vi "Sub01_CommandBuilder.vi"(8 "error in (no error)":errorcluster, 9 "CommandInfo":T1={"RedBall"={"Min"={"G"=0, "B"=0, "R"=160}, "Max"={"G"=160, "B"=160, "R"=255}}, "YellowBall"={"Min"={"G"=140, "B"=0, "R"=140}, "Max"={"G"=255, "B"=175, "R"=255}}, "WhiteBall"={"Min"={"G"=100, "B"=100, "R"=100}, "Max"={"G"=255, "B"=255, "R"=255}}, "BallDiameter"=11, "BackGround"={"Min"={"G"=91, "B"=202, "R"=39}, "Max"={"G"=116, "B"=255, "R"=62}}, "Border"={"Min"={"G"=0, "B"=121, "R"=0}, "Max"={"G"=42, "B"=126, "R"=14}}}, 10 "filenames":string[](array[string]), 11 "path in":path) -> (0 "error out":errorcluster, 3 "String":string)   [LabVIEW 2019]
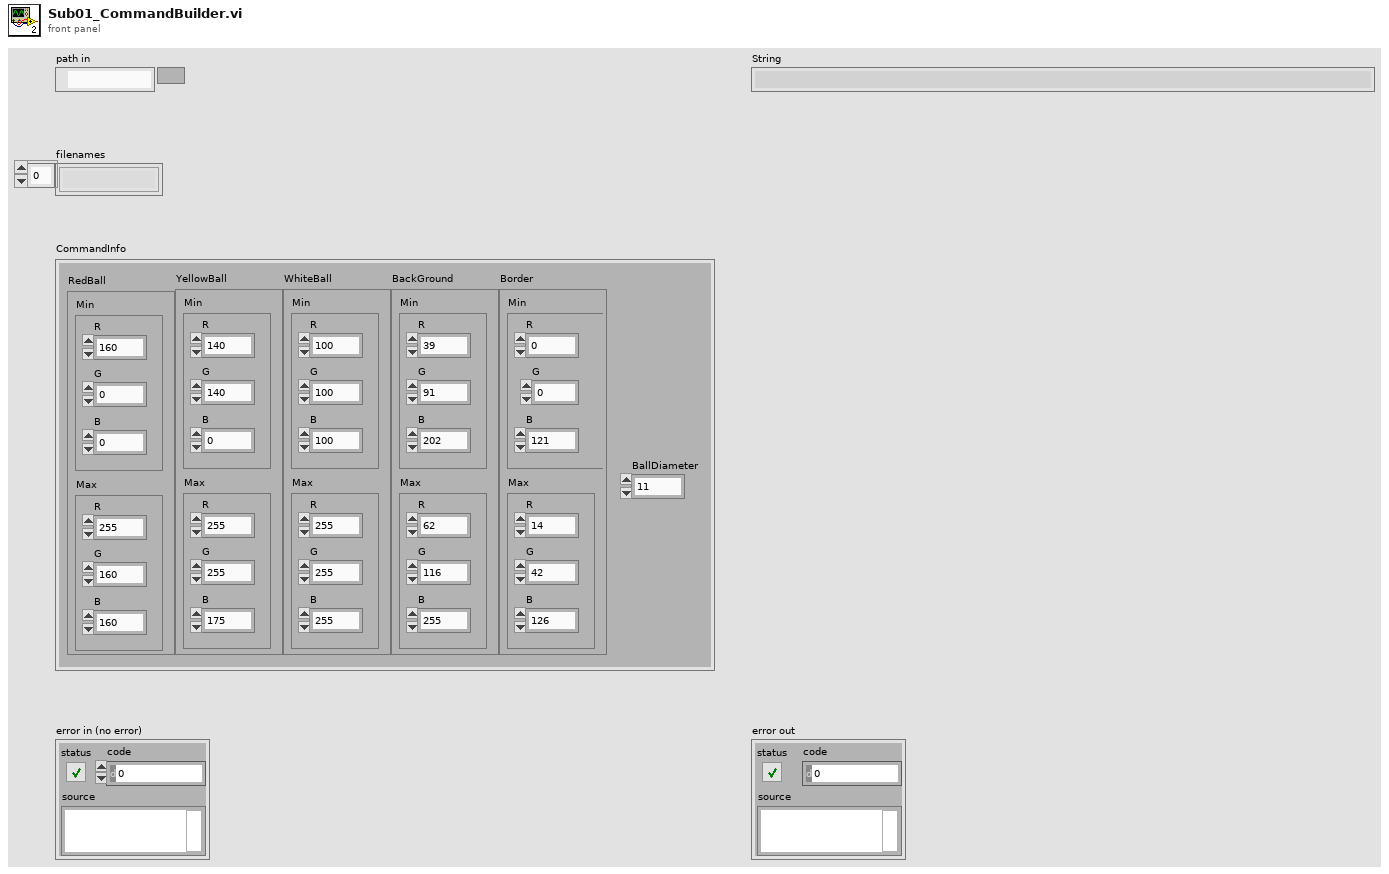
[diagram p1: front panel]
types:
  T1 = cluster{"RedBall":cluster{"Min":cluster{"G":u32, "B":u32, "R":u32}, "Max":cluster{"G":u32, "B":u32, "R":u32}}, "YellowBall":cluster{"Min":cluster{"G":u32, "B":u32, "R":u32}, "Max":cluster{"G":u32, "B":u32, "R":u32}}, "WhiteBall":cluster{"Min":cluster{"G":u32, "B":u32, "R":u32}, "Max":cluster{"G":u32, "B":u32, "R":u32}}, "BallDiameter":u32, "BackGround":cluster{"Min":cluster{"G":u32, "B":u32, "R":u32}, "Max":cluster{"G":u32, "B":u32, "R":u32}}, "Border":cluster{"Min":cluster{"G":u32, "B":u32, "R":u32}, "Max":cluster{"G":u32, "B":u32, "R":u32}}}
  T2 = typedef "imagedata.ctl" = cluster{"image type":i32, "image depth":i32, "image":u8[], "mask":u8[], "colors":u32[], "Rectangle":cluster{"left":i16, "top":i16, "right":i16, "bottom":i16}}
  T3 = cluster{"Min":cluster{"G":u32, "B":u32, "R":u32}, "Max":cluster{"G":u32, "B":u32, "R":u32}}
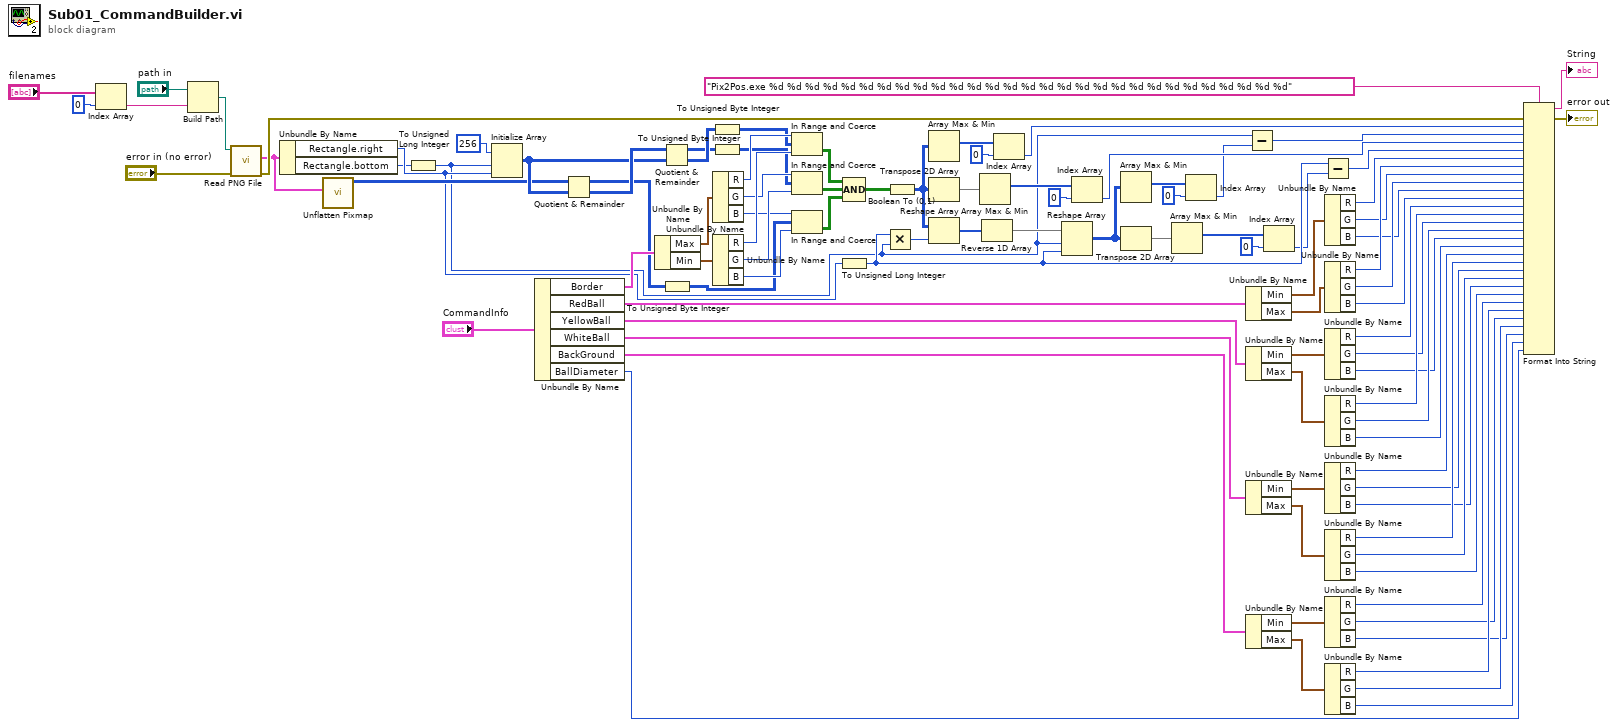
[diagram p0: block diagram]
diagram:
  n1 = Index Array(array="filenames", index=0) -> (element=w32:string)
  n2 = Build Path(base path="path in", name or relative path=w32) -> (appended path=w93:path)
  n3 = call <vilib>:"Read PNG File.vi"("error in (no error)"="error in (no error)", "path to PNG file"=w93) -> ("error out"=w94:errorcluster, "image data"=w30:T2)  [unwired: 7 in, 1 out]
  n4 = Unbundle By Name(w30) -> ("Rectangle.right"=w18:i16, "Rectangle.bottom"=w17:i16)
  n5 = call <vilib>:"Unflatten Pixmap.vi"("image data"=w30) -> ("24-bit pixmap"=w31:u32[][])  [unwired: 4 in, 6 out]
  n6 = To Unsigned Long Integer(number=w17) -> (unsigned 32bit integer=w7:u32)
  n7 = Initialize Array(u32 256 ("element"), w7, w18) -> (w37:u32[][])
  n8 = Unbundle By Name("CommandInfo") -> ("Border"=w50:T3, "RedBall"=w88:T3, "YellowBall"=w81:T3, "WhiteBall"=w80:T3, "BackGround"=w71:T3, "BallDiameter"=w49:u32)
  n9 = Quotient & Remainder(x=w31, y=w37) -> (x-y*floor(x/y)=w44:u32[][], floor(x/y)=w47:u32[][])
  n10 = Unbundle By Name(w50) -> ("Max"=w52:cluster{"G":u32, "B":u32, "R":u32}, "Min"=w51:cluster{"G":u32, "B":u32, "R":u32})
  n11 = Quotient & Remainder(x=w47, y=w37) -> (x-y*floor(x/y)=w45:u32[][], floor(x/y)=w46:u32[][])
  n12 = To Unsigned Byte Integer(number=w44) -> (unsigned 8bit integer=w36:u8[][])
  n13 = To Unsigned Byte Integer(number=w46) -> (unsigned 8bit integer=w34:u8[][])
  n14 = To Unsigned Byte Integer(number=w45) -> (unsigned 8bit integer=w35:u8[][])
  n15 = Unbundle By Name(w52) -> ("R"=w43:u32, "G"=w41:u32, "B"=w39:u32)
  n16 = Unbundle By Name(w51) -> ("R"=w42:u32, "G"=w40:u32, "B"=w38:u32)
  n17 = In Range and Coerce(upper limit=w43, x=w34, lower limit=w42) -> (In Range?=w29:bool[][])  [unwired: 1 out]
  n18 = In Range and Coerce(upper limit=w41, x=w35, lower limit=w40) -> (In Range?=w28:bool[][])  [unwired: 1 out]
  n19 = In Range and Coerce(upper limit=w39, x=w36, lower limit=w38) -> (In Range?=w27:bool[][])  [unwired: 1 out]
  n20 = To Unsigned Long Integer(number=w18) -> (unsigned 32bit integer=w8:u32)
  n21 = Compound Arithmetic op=AND(w29, w28, w27) -> (w26:bool[][])
  n22 = Multiply(x=w8, y=w7) -> (x*y=w25:u32)
  n23 = Boolean To (0,1)(Boolean=w26) -> (0, 1=w20:i16[][])
  n24 = Array Max & Min(array=w20) -> (max index (indices)=w12:i32[])  [unwired: 3 out]
  n25 = Transpose 2D Array(2D array=w20) -> (transposed array=w23:i16[][])
  n26 = Reshape Array(w20, w25) -> (w21:i16[])
  n27 = Array Max & Min(array=w23) -> (max index (indices)=w11:i32[])  [unwired: 3 out]
  n28 = Reverse 1D Array(array=w21) -> (reversed array=w24:i16[])
  n29 = Index Array(array=w12, index=0) -> (element=w6:i32)
  n30 = Reshape Array(w24, w7, w8) -> (w19:i16[][])
  n31 = Index Array(array=w11, index=0) -> (element=w5:i32)
  n32 = Array Max & Min(array=w19) -> (max index (indices)=w9:i32[])  [unwired: 3 out]
  n33 = Transpose 2D Array(2D array=w19) -> (transposed array=w22:i16[][])
  n34 = Array Max & Min(array=w22) -> (max index (indices)=w10:i32[])  [unwired: 3 out]
  n35 = Index Array(array=w9, index=0) -> (element=w4:i32)
  n36 = Unbundle By Name(w88) -> ("Min"=w87:cluster{"G":u32, "B":u32, "R":u32}, "Max"=w86:cluster{"G":u32, "B":u32, "R":u32})
  n37 = Unbundle By Name(w81) -> ("Min"=w85:cluster{"G":u32, "B":u32, "R":u32}, "Max"=w84:cluster{"G":u32, "B":u32, "R":u32})
  n38 = Unbundle By Name(w80) -> ("Min"=w83:cluster{"G":u32, "B":u32, "R":u32}, "Max"=w82:cluster{"G":u32, "B":u32, "R":u32})
  n39 = Unbundle By Name(w71) -> ("Min"=w73:cluster{"G":u32, "B":u32, "R":u32}, "Max"=w72:cluster{"G":u32, "B":u32, "R":u32})
  n40 = Subtract(x=w7, y=w4) -> (x-y=w3:u32)
  n41 = Index Array(array=w10, index=0) -> (element=w2:i32)
  n42 = Subtract(x=w8, y=w2) -> (x-y=w1:u32)
  n43 = Unbundle By Name(w87) -> ("R"=w79:u32, "G"=w77:u32, "B"=w75:u32)
  n44 = Unbundle By Name(w86) -> ("R"=w78:u32, "G"=w76:u32, "B"=w74:u32)
  n45 = Unbundle By Name(w85) -> ("R"=w70:u32, "G"=w68:u32, "B"=w66:u32)
  n46 = Unbundle By Name(w84) -> ("R"=w69:u32, "G"=w67:u32, "B"=w65:u32)
  n47 = Unbundle By Name(w83) -> ("R"=w64:u32, "G"=w62:u32, "B"=w60:u32)
  n48 = Unbundle By Name(w82) -> ("R"=w63:u32, "G"=w61:u32, "B"=w59:u32)
  n49 = Unbundle By Name(w73) -> ("R"=w58:u32, "G"=w56:u32, "B"=w54:u32)
  n50 = Unbundle By Name(w72) -> ("R"=w57:u32, "G"=w55:u32, "B"=w53:u32)
  n51 = Format Into String(format string="Pix2Pos.exe %d %d %d %d %d %d %d %d %d %d %d %d %d %d %d %d %d %d %d %d %d %d %d %d %d %d %d %d %d", error in=w94, w6, w3, w5, w1, w79, w78, w77, w76, w75, w74, w70, w69, w68, w67, w66, w65, w64, w63, w62, w61, w60, w59, w58, w57, w56, w55, w54, w53, w49) -> (resulting string=→"String":string, error out=→"error out":errorcluster)  [unwired: 1 in]
